vi "create Variable.vi"(0 "Variable Manager Trigger Event":refnum<class "HGF_Event.lvclass">, 2 "Variable name":string, 4 "timeout":i32, 5 "error in (no error)":errorcluster) -> (16 "Variable":refnum<k21>, 17 "create Variable timed out":bool, 19 "error out":errorcluster)   [LabVIEW 2009, in "MoAgSy.lvlib"]
uses:
  MoAgSy.lvlib
  HGF_BaseClasses/HGF_Event/HGF_Event.lvclass
  HGF_SV/HGF_SVFactory/HGF_SVFactory.lvclass
  HGF_BaseClasses/HGF_TriggeredEvent/HGF_TriggeredEvent.lvclass
  HGF_SV/Visitors/HGF_SVVarManVisitor_create/HGF_SVVarManVisitor_create.lvclass
  HGF_BaseClasses/HGF_Factory/HGF_Factory.lvclass
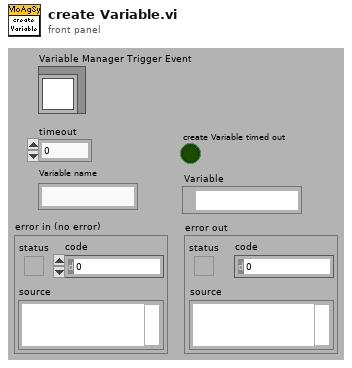
[diagram p1: front panel]
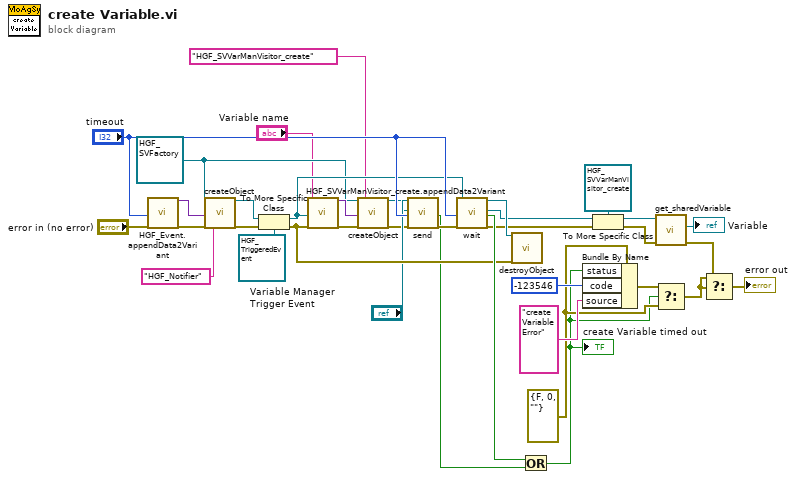
[diagram p0: block diagram]
diagram:
  w33 = errorcluster {"status"=FALSE, "code"=0, "source"=""} ("error out")
  w11 = refnum<class "HGF_SVFactory.lvclass"> refnum ("HGF_SV.lvlib:HGF_SVFactory.lvclass")
  n1 = call "HGF_Event.appendData2Variant.vi"("timeout in ms (-1)"="timeout", "error in (no error)"="error in (no error)") -> ("dup initData"=w9:variant, "error out"=w10:errorcluster)  [unwired: 16 in]
  n2 = call "createObject.vi"("HGF_Factory"=w11, "initializationData"=w9, "error in (no error)"=w10, "className"="HGF_Notifier") -> ("HGF_Object"=w14:refnum<class "HGF_Factory.lvclass">, "error out"=w16:errorcluster)  [unwired: 1 in, 13 out]
  n3 = To More Specific Class(target class=refnum<class "HGF_TriggeredEvent.lvclass"> refnum ("DSC Exception"), reference=w14, error in=w16) -> (specific class reference=w18:refnum<class "HGF_TriggeredEvent.lvclass">, error out=w32:errorcluster)
  n4 = call "HGF_SVVarManVisitor_create.appendData2Variant.vi"("SV Name"="Variable name", "return-to Event"=w18, "error in"=w32) -> ("dup variant"=w17:variant, "error out"=w19:errorcluster)  [unwired: 15 in]
  n5 = call "createObject.vi"("HGF_Factory"=w11, "initializationData"=w17, "error in (no error)"=w19, "className"="HGF_SVVarManVisitor_create") -> ("HGF_Object"=w20:refnum<class "HGF_Factory.lvclass">, "error out"=w21:errorcluster)  [unwired: 1 in, 13 out]
  n6 = call-dynamic "send.vi"("HGF_Event"="Variable Manager Trigger Event", "Object"=w20, "timeout in ms (-1)"="timeout", "error in (no error)"=w21) -> ("timed out?"=w4:bool, "error out"=w22:errorcluster)  [unwired: 13 in, 1 out]
  n7 = call-dynamic "wait.vi"("HGF_Event"=w18, "msTimeout (-1)"="timeout", "error in (no error)"=w22) -> ("dup HGF_Event"=w31:refnum<class "HGF_TriggeredEvent.lvclass">, "Object"=w25:refnum<class>, "timed out"=w34:bool, "error out"=w27:errorcluster)  [unwired: 13 in]
  n8 = call "destroyObject.vi"("HGF_Factory"=w31, "error in (no error)"=w32) -> ()  [unwired: 17 in, 1 out]
  n9 = Or(x=w34, y=w4) -> (x .or. y?=w5:bool)
  "create Variable timed out" <- w5
  n10 = Bundle By Name(cluster=w33, "status"=w5, "code"=-123546, "source"="create  Variable Error") -> (w8:errorcluster)
  n11 = To More Specific Class(target class=refnum<class "HGF_SVVarManVisitor_create.lvclass"> refnum ("HGF_SV.lvlib:HGF_SVVarManVisitor_create.lvclass"), reference=w25, error in=w27) -> (specific class reference=w28:refnum<class "HGF_SVVarManVisitor_create.lvclass">, error out=w29:errorcluster)
  n12 = call "get_sharedVariable.vi"("error in (no error)"=w29, "HGF_SVVarManVisitor_create in"=w28) -> ("error out"=w1:errorcluster, "shared variable"=→"Variable":refnum<k21>)  [unwired: 7 in, 1 out]
  n13 = Select(t=w8, s=w5, f=w33) -> (s? t:f=w2:errorcluster)
  n14 = Select(t=w2, s=w2, f=w1) -> (s? t:f=→"error out":errorcluster)
